vi "From JSON.vi"(8 "error in (no error)":errorcluster, 10 "JSON":string, 11 "Double Float in":refnum<class "AbsFunc_Two Term_DBL.lvclass">) -> (0 "error out":errorcluster, 2 "Remaining JSON":string, 3 "Double Float out":refnum<class "AbsFunc_Two Term_DBL.lvclass">)   [LabVIEW 2021, in "AbsFunc_Two Term_DBL.lvclass"]
uses:
  AbsFunc_Two Term_DBL.lvclass
  Abs_Types/Double Float/Abs_Double Float.lvclass
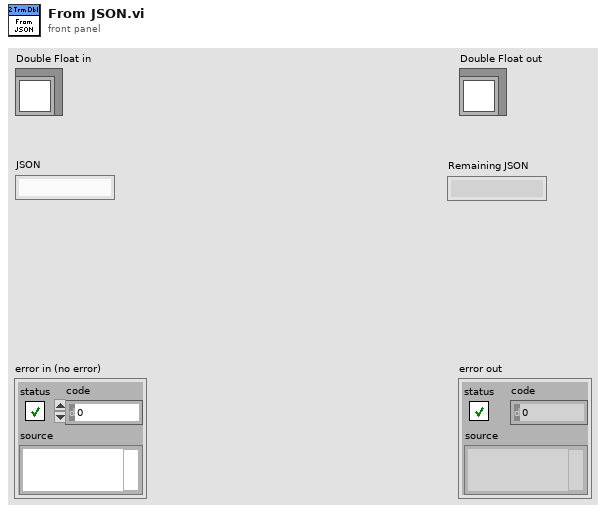
[diagram p1: front panel]
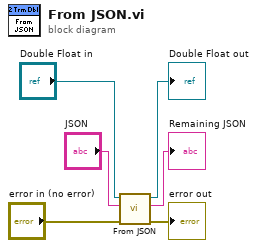
[diagram p0: block diagram]
diagram:
  n1 = call-parent "From JSON.vi"("error in (no error)"="error in (no error)", "JSON"="JSON", "Double Float in"="Double Float in") -> ("error out"=→"error out":errorcluster, "Remaining JSON"=→"Remaining JSON":string, "Double Float out"=→"Double Float out":refnum<class "AbsFunc_Two Term_DBL.lvclass">)  [unwired: 6 in]
